vi "GV_YscaleUpdateMenu.vi"(8 "error in (no error)":errorcluster, 11 "Gviewer in":refnum<class "Gviewer.lvclass">) -> (0 "error out":errorcluster, 3 "Gviewer out":refnum<class "Gviewer.lvclass">)   [LabVIEW 2020, in "Sgraph_lib_V1.lvlib" / "Gviewer.lvclass"]
doc: "Set the Y-scale menu items ON/OFF based upon Y-scales present or not"
uses:
  Gviewer.lvclass
  Gviewer.lvclass/Gviewer.ctl
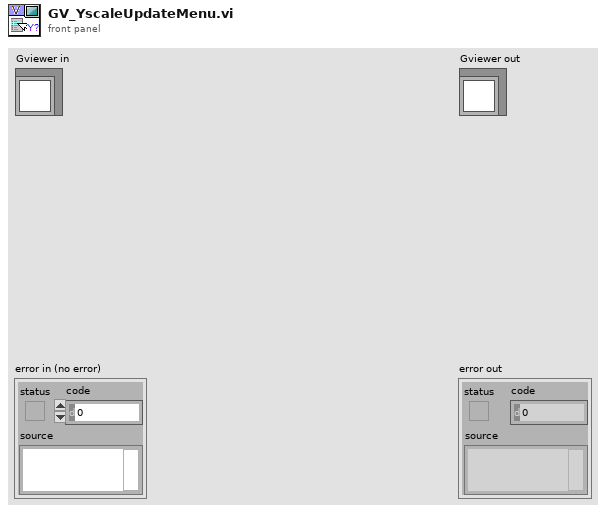
[diagram p1: front panel]
types:
  T1 = typedef "Sgraph_lib_V1.lvlib/Gviewer.lvclass/YgraphDef.ctl" = cluster{"Plot":i32, "X(%)":dbl}
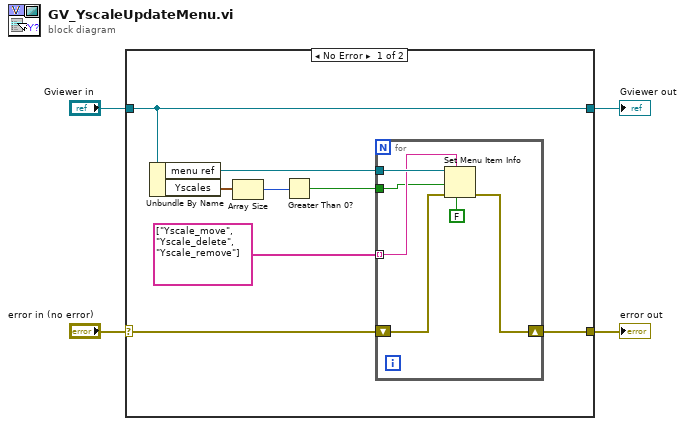
[diagram p0: block diagram]
diagram:
  n1 = case shown="No Error" "error in (no error)" {
    selector: "error in (no error)" -> [w6 w20]
    tunnel: [w5 w20] -> w3
    tunnel: [w12 w19] -> w1
    tunnel: "Gviewer in" -> [w12 w19]
    frame No Error {
      n2 = Unbundle By Name(w12) -> ("menu ref"=w8:refnum<k9>, "Yscales"=w11:T1[])
      n3 = Array Size(array=w11) -> (size(s)=w9:i32)
      n4 = Greater Than 0?(x=w9) -> (x > 0?=w7:bool)
      n5 = for {
        tunnel: string[] ["Yscale_move", "Yscale_delete", "Yscale_remove"] -> [w17] mode=indexing
        tunnel: w8 -> [w18]
        tunnel: w7 -> [w15]
        shift-right: [w13] -> w5
        shift-left: w6 -> [w14]
        n6 = Set Menu Item Info(6:FALSE ("checked"), 7:w17, 8:w14, 9:w15, 11:w18) -> (0:w13:errorcluster)  [unwired: 2 in, 1 out]
      }
    }
    frame Error {
    }
  }
  "error out" <- w3
  "Gviewer out" <- w1
